vi "Array Max and Min.vi"() -> ()   [LabVIEW 2014]
panel:
  out "最小值索引":i32[](array[numeric])
  out "最小值":i32
  out "最大值索引":i32[](array[numeric])
  out "最大值":i32
  out "最小值":i32
  out "最小值索引":i32
  out "最大值索引":i32
  out "最大值":i32
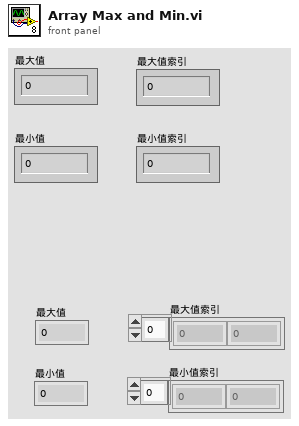
[diagram p1: front panel]
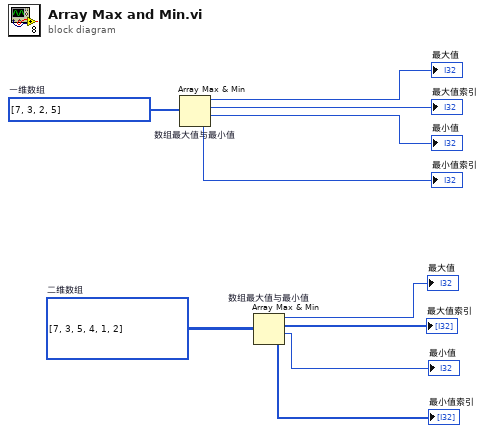
[diagram p0: block diagram]
diagram:
  w9 = i32[][] [[7, 3, 5], [4, 1, 2]]  # 二维数组
  w10 = i32[] [7, 3, 2, 5]  # 一维数组
  n1 = Array Max & Min "数组最大值与最小值"(array=w10) -> (max value=→"最大值":i32, max index (indices)=→"最大值索引":i32, min value=→"最小值":i32, min index (indices)=→"最小值索引":i32)
  n2 = Array Max & Min "数组最大值与最小值"(array=w9) -> (max value=→"最大值":i32, max index (indices)=→"最大值索引":i32[], min value=→"最小值":i32, min index (indices)=→"最小值索引":i32[])
